vi "neverrest-motor-encoder.vi"   [LabVIEW 2012, in "Testing.lvrbt"]
uses:
  Testing.lvrbt
  <vilib>/NXT/LegoClasses/BrickReference/BrickReference.lvclass
  <vilib>/NXT/Subs/LVHSConnector.ctl
  <vilib>/NXT/NXTIO Xnodes/NXTIOXNode/NXTIO.xnode
  <vilib>/NXT/Hardware/Plugins/Open Port/OpenPortAddress.ctl
  <vilib>/NXT/NXTIO Xnodes/AddressXNode/NXTIOAddress.xnode
types:
  T1 = typedef "OpenPortAddress.ctl" = i32
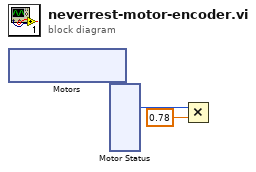
[diagram p0: block diagram]
diagram:
  n1 = xnode "Motors"() -> ("Motor"=w3:T1)
  n2 = xnode "Motor Status"("Motors"=w3) -> ("Position 1"=w2:i32)  [unwired: 1 in, 2 out]
  n3 = Multiply(x=w2, y=0.78) -> ()  [unwired: 1 out]
